vi "RT Main.vi"   [LabVIEW 2017]
doc: "This template is for the Queued Message Handler design pattern.\n\nThe Event Handling Loop generates messages based on user interface actions.\n\nThe Message Handling Loop processes messages generated by the Event Handling Loop, or by other messages. The messages are string values, so new messages can be added easily to the Message Cases case structure in the Message Handling Loop. Each message cluster can also provide an optional value for Message Data, which is a variant that can be converted to whatever message-specific data is required."
uses:
  controls/Functional Global Operation.ctl
  controls/Control State.ctl
  controls/Raw Values.ctl
  controls/Control Configuration.ctl
  Globals/Global - RT Stream Connections.vi
  Globals/Global - Configuration Options.vi
  support/Message Queue/Message Queue.lvlib
  <vilib>/nisyscfg/nisyscfg.lvlib
types:
  T1 = typedef "Functional Global Operation.ctl" = enum16{"Initialize", "Read", "Write"}
  T2 = typedef "Control State.ctl" = enum16{"Safe State", "Manual", "Control (PID)"}
  T3 = typedef "Raw Values.ctl" = cluster{"Channel 0":dbl, "Channel 1":dbl, "Channel 2":dbl, "Channel 3":dbl}
  T4 = typedef "Control Configuration.ctl" = cluster{"PID Gains":cluster{"proportional gain (Kc)":dbl, "integral gain (Kc*Ts/Ti)":dbl, "derivative gain (Kc*Td/Ts)":dbl}, "Output Range":cluster{"output high":dbl, "output low":dbl}}
  T5 = typedef "All Control Configuration Values.ctl" = cluster{"Control State":T2, "Setpoints":T3, "Manual Values":T3, "Control Configurations":T4[]}
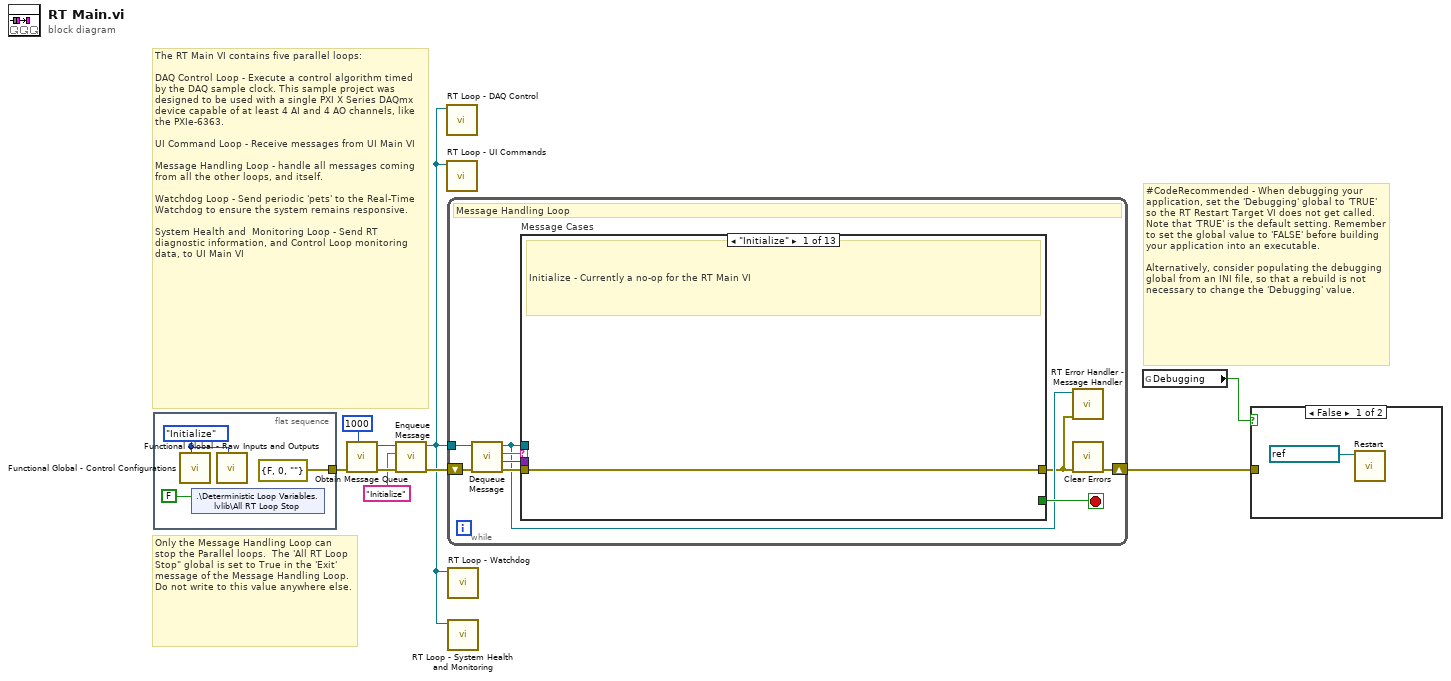
[diagram p0: block diagram]
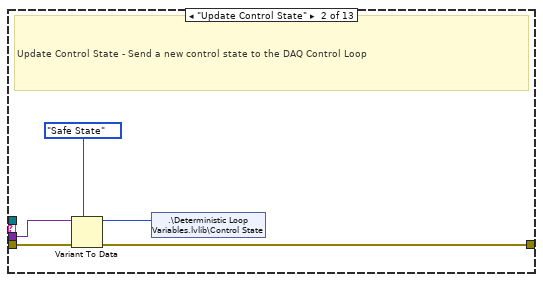
[diagram p3: hidden frame]
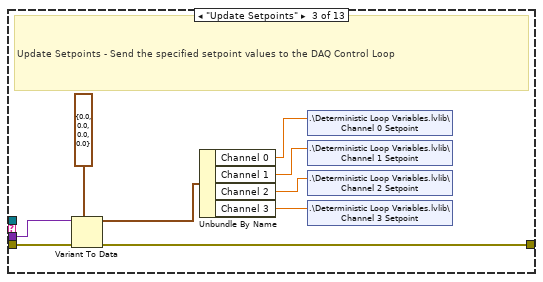
[diagram p4: hidden frame]
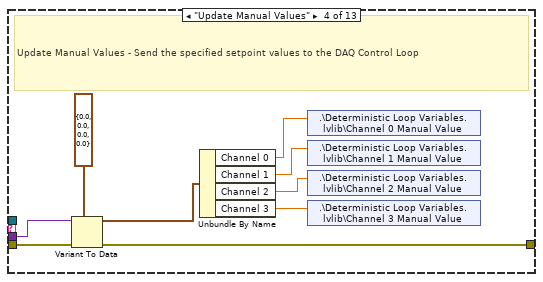
[diagram p5: hidden frame]
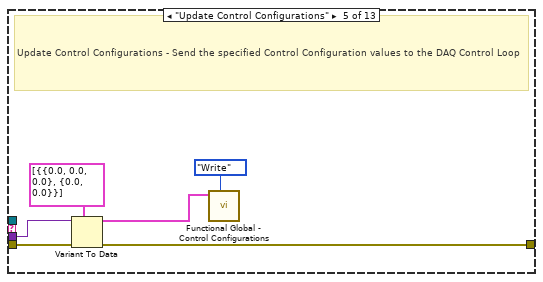
[diagram p6: hidden frame]
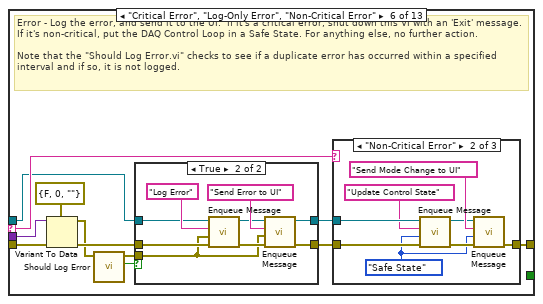
[diagram p7: hidden frame]
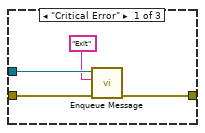
[diagram p9: hidden frame]
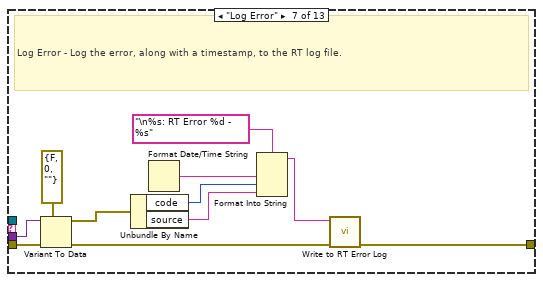
[diagram p11: hidden frame]
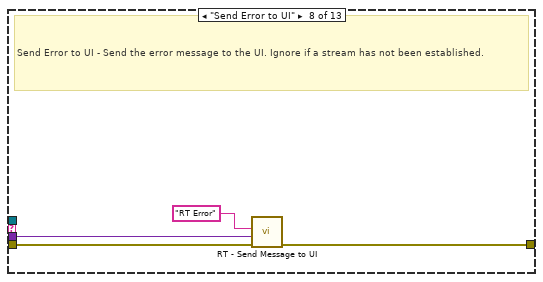
[diagram p12: hidden frame]
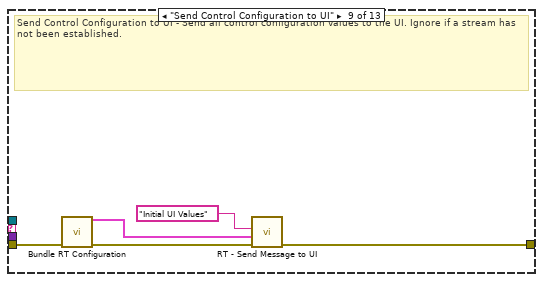
[diagram p13: hidden frame]
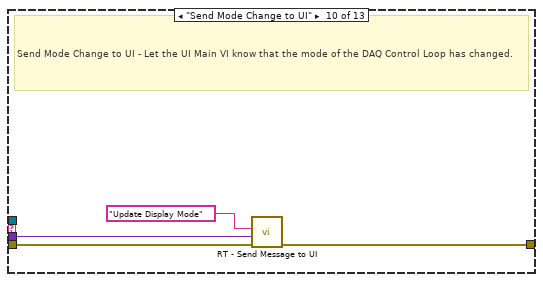
[diagram p14: hidden frame]
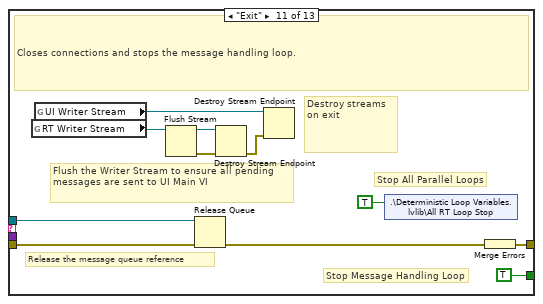
[diagram p15: hidden frame]
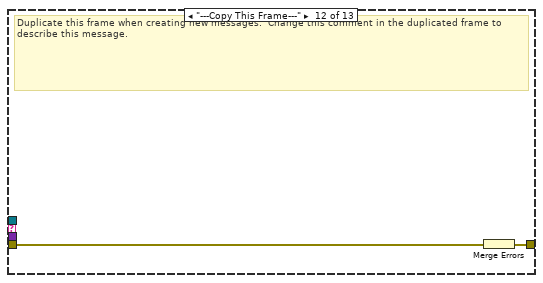
[diagram p16: hidden frame]
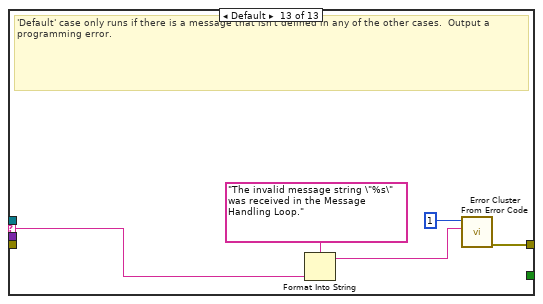
[diagram p17: hidden frame]
diagram:
  # "#CodeRecommended - When debugging your application, set the 'Debugging' global to 'TRUE' so the RT Restart Target VI does not get called.  Note that 'TRUE' is the default setting. Remember to set the global value to 'FALSE' before building your application into an executable.\n\nAlternatively, consider populating the debugging global from an INI file, so that a rebuild is not necessary to change the 'Debugging' value."
  # "The RT Main VI contains five parallel loops:\n\nDAQ Control Loop - Execute a control algorithm timed by the DAQ sample clock. This sample project was designed to be used with a single PXI X Series DAQmx device capable of at least 4 AI and 4 AO channels, like the PXIe-6363.\n\nUI Command Loop - Receive messages from UI Main VI\n\nMessage Handling Loop - handle all messages coming from all the other loops, and itself.\n\nWatchdog Loop - Send periodic 'pets' to the Real-Time Watchdog to ensure the system remains responsive.\n\nSystem Health and  Monitoring Loop - Send RT diagnostic information, and Control Loop monitoring data, to UI Main VI"
  # "Only the Message Handling Loop can stop the Parallel loops.  The 'All RT Loop Stop\" global is set to True in the 'Exit' message of the Message Handling Loop.  Do not write to this value anywhere else."
  n1 = flat-sequence {
    tunnel: [errorcluster {"status"=FALSE, "code"=0, "source"=""} ("error constant")] -> w4
    frame #0 {
      w10 = Functional_Global_Operation."Initialize" ("Functional Global Operation (Read)")
      n2 = call "Functional Global - Control Configurations.vi"("Functional Global Operation (Read)"=w10) -> ()  [unwired: 10 in, 1 out]
      n3 = shared-variable ".\\Deterministic Loop Variables.lvlib\\All RT Loop Stop"(FALSE) -> ()  [unwired: 1 in, 1 out]
      n4 = call "Functional Global - Raw Inputs and Outputs.vi"("Functional Global Operation (Read)"=w10) -> ()  [unwired: 9 in, 2 out]
    }
  }
  n5 = call "Obtain Message Queue.vi"("max queue size (-1, unlimited)"=1000, "error in (no error)"=w4) -> ("error out"=w9:errorcluster, "Message Queue"=w8:refnum<queue>)  [unwired: 8 in]
  n6 = call "Enqueue Message.vi"("error in (no error)"=w9, "Message"="Initialize", "Message Queue"=w8) -> ("error out"=w6:errorcluster, "dup Message Queue"=w2:refnum<queue>)  [unwired: 7 in]
  n7 = call "RT Loop - DAQ Control.vi"("Message Queue"=w2) -> ()  [unwired: 11 in]
  n8 = call "RT Loop - UI Commands.vi"("Message Queue"=w2) -> ()  [unwired: 11 in]
  n9 = while {
    tunnel: w2 -> [w16]
    shift-right: [w14] -> w3
    shift-left: w6 -> [w20]
    stop <- w21 stop-if-true
    # "Message Handling Loop"
    n10 = call "Dequeue Message.vi"("error in (no error)"=w20, "Message Queue"=w16) -> ("error out"=w19:errorcluster, "Message Data"=w17:variant, "Message"=w18:string, "dup Message Queue"=w15:refnum<queue>)  [unwired: 6 in]
    n11 = case "Message Cases" shown="\"Initialize\"" w18 {
      selector: w18 -> [_ _ _ _ _ w61 _ _ _ _ _ _ w128]
      tunnel: w15 -> [_ _ _ _ _ w55 _ _ _ _ w122 _ _]
      tunnel: w19 -> [w22 w27 w36 w45 w51 w59 w98 w102 w107 w111 w118 w124 _]
      tunnel: [w22 w24 w32 w41 w48 w60 w89 w99 w103 w110 w119 w123 w126] -> w13
      tunnel: [_ _ _ _ _ _ _ _ _ _ TRUE _ _] -> w21
      tunnel: w17 -> [_ w26 w35 w44 w50 w58 w97 w101 _ w109 _ _ _]
      frame "Initialize" {
        # "Initialize - Currently a no-op for the RT Main VI"
      }
      frame "Update Control State" {
        # "Update Control State - Send a new control state to the DAQ Control Loop"
        n12 = Variant To Data(error in=w27, type=Control_State."Safe State" ("FPGA State"), Variant=w26) -> (data=w23:T2, error out=w24:errorcluster)
        n13 = shared-variable ".\\Deterministic Loop Variables.lvlib\\Control State"(w23) -> ()  [unwired: 1 in, 1 out]
      }
      frame "Update Setpoints" {
        # "Update Setpoints - Send the specified setpoint values to the DAQ Control Loop"
        n14 = Variant To Data(error in=w36, type=T3 {"Channel 0"=0.0, "Channel 1"=0.0, "Channel 2"=0.0, "Channel 3"=0.0} ("Raw Values"), Variant=w35) -> (data=w33:T3, error out=w32:errorcluster)
        n15 = Unbundle By Name(w33) -> ("Channel 0"=w28:dbl, "Channel 1"=w29:dbl, "Channel 2"=w30:dbl, "Channel 3"=w31:dbl)
        n16 = shared-variable ".\\Deterministic Loop Variables.lvlib\\Channel 0 Setpoint"(w28) -> ()  [unwired: 1 in, 1 out]
        n17 = shared-variable ".\\Deterministic Loop Variables.lvlib\\Channel 1 Setpoint"(w29) -> ()  [unwired: 1 in, 1 out]
        n18 = shared-variable ".\\Deterministic Loop Variables.lvlib\\Channel 2 Setpoint"(w30) -> ()  [unwired: 1 in, 1 out]
        n19 = shared-variable ".\\Deterministic Loop Variables.lvlib\\Channel 3 Setpoint"(w31) -> ()  [unwired: 1 in, 1 out]
      }
      frame "Update Manual Values" {
        # "Update Manual Values - Send the specified setpoint values to the DAQ Control Loop"
        n20 = Variant To Data(error in=w45, type=T3 {"Channel 0"=0.0, "Channel 1"=0.0, "Channel 2"=0.0, "Channel 3"=0.0} ("Raw Values"), Variant=w44) -> (data=w42:T3, error out=w41:errorcluster)
        n21 = Unbundle By Name(w42) -> ("Channel 0"=w37:dbl, "Channel 1"=w38:dbl, "Channel 2"=w39:dbl, "Channel 3"=w40:dbl)
        n22 = shared-variable ".\\Deterministic Loop Variables.lvlib\\Channel 0 Manual Value"(w37) -> ()  [unwired: 1 in, 1 out]
        n23 = shared-variable ".\\Deterministic Loop Variables.lvlib\\Channel 1 Manual Value"(w38) -> ()  [unwired: 1 in, 1 out]
        n24 = shared-variable ".\\Deterministic Loop Variables.lvlib\\Channel 2 Manual Value"(w39) -> ()  [unwired: 1 in, 1 out]
        n25 = shared-variable ".\\Deterministic Loop Variables.lvlib\\Channel 3 Manual Value"(w40) -> ()  [unwired: 1 in, 1 out]
      }
      frame "Update Control Configurations" {
        # "Update Control Configurations - Send the specified Control Configuration values to the DAQ Control Loop"
        n26 = Variant To Data(error in=w51, type=T4[] [{"PID Gains"={"proportional gain (Kc)"=0.0, "integral gain (Kc*Ts/Ti)"=0.0, "derivative gain (Kc*Td/Ts)"=0.0}, "Output Range"={"output high"=0.0, "output low"=0.0}}], Variant=w50) -> (data=w47:T4[], error out=w48:errorcluster)
        n27 = call "Functional Global - Control Configurations.vi"("Functional Global Operation (Read)"=Functional_Global_Operation."Write", "Control Configurations in"=w47) -> ()  [unwired: 9 in, 1 out]
      }
      frame "Critical Error", "Log-Only Error", "Non-Critical Error" {
        # "Error - Log the error, and send it to the UI.  If it's a critical error, shut down this VI with an 'Exit' message. If it's non-critical, put the DAQ Control Loop in a Safe State. For anything else, no further action.\n\nNote that the \"Should Log Error.vi\" checks to see if a duplicate error has occurred within a specified interval and if so, it is not logged."
        n28 = Variant To Data(error in=w59, type=errorcluster {"status"=FALSE, "code"=0, "source"=""} ("error out"), Variant=w58) -> (data=w53:errorcluster, error out=w56:errorcluster)
        n29 = call "Should Log Error.vi"("error to report"=w53) -> ("Should Log Error?"=w54:bool, "dup error to report"=w52:errorcluster)  [unwired: 9 in]
        n30 = case shown="True" w54 {
          tunnel: [w65 w72] -> w63
          tunnel: [w64 w71] -> w62
          tunnel: w55 -> [w64 w70]
          tunnel: w56 -> [w65 w67]
          tunnel: w52 -> [_ w66]
          frame False {
          }
          frame True {
            n31 = call "Enqueue Message.vi"("error in (no error)"=w67, "Message Data"=w66, "Message"="Log Error", "Message Queue"=w70) -> ("error out"=w68:errorcluster, "dup Message Queue"=w69:refnum<queue>)  [unwired: 6 in]
            n32 = call "Enqueue Message.vi"("error in (no error)"=w68, "Message Data"=w66, "Message"="Send Error to UI", "Message Queue"=w69) -> ("error out"=w72:errorcluster, "dup Message Queue"=w71:refnum<queue>)  [unwired: 6 in]
          }
        }
        n33 = case shown="\"Non-Critical Error\"" w61 {
          tunnel: w63 -> [w78 w86 w87]
          tunnel: w62 -> [w76 w85 _]
          tunnel: [w77 w82 w87] -> w60
          frame "Critical Error" {
            n34 = call "Enqueue Message.vi"("error in (no error)"=w78, "Message"="Exit", "Message Queue"=w76) -> ("error out"=w77:errorcluster)  [unwired: 7 in, 1 out]
          }
          frame "Non-Critical Error" {
            w79 = Control_State."Safe State" ("FPGA State")
            n35 = call "Enqueue Message.vi"("error in (no error)"=w86, "Message Data"=w79, "Message"="Update Control State", "Message Queue"=w85) -> ("error out"=w83:errorcluster, "dup Message Queue"=w80:refnum<queue>)  [unwired: 6 in]
            n36 = call "Enqueue Message.vi"("error in (no error)"=w83, "Message Data"=w79, "Message"="Send Mode Change to UI", "Message Queue"=w80) -> ("error out"=w82:errorcluster)  [unwired: 6 in, 1 out]
          }
          frame Default {
          }
        }
      }
      frame "Log Error" {
        # "Log Error - Log the error, along with a timestamp, to the RT log file."
        n37 = Variant To Data(error in=w98, type=errorcluster {"status"=FALSE, "code"=0, "source"=""} ("error constant"), Variant=w97) -> (data=w92:errorcluster, error out=w95:errorcluster)
        n38 = Unbundle By Name(w92) -> ("code"=w91:i32, "source"=w90:string)
        n39 = Format Date/Time String() -> (date/time string=w93:string)  [unwired: 3 in]
        n40 = Format Into String(format string="\n%s: RT Error %d - %s", w93, w91, w90) -> (resulting string=w88:string)  [unwired: 2 in, 1 out]
        n41 = call "Write to RT Error Log.vi"("error in (no error)"=w95, "Log Entry"=w88) -> ("error out"=w89:errorcluster)  [unwired: 9 in]
      }
      frame "Send Error to UI" {
        # "Send Error to UI - Send the error message to the UI. Ignore if a stream has not been established."
        n42 = call "RT - Send Message to UI.vi"("error in (no error)"=w102, "Message Data"=w101, "Message"="RT Error") -> ("error out"=w99:errorcluster)  [unwired: 8 in]
      }
      frame "Send Control Configuration to UI" {
        # "Send Control Configuration to UI - Send all control configuration values to the UI. Ignore if a stream has not been established."
        n43 = call "Bundle RT Configuration.vi"("error in (no error)"=w107) -> ("error out"=w106:errorcluster, "All Control Configuration Values"=w105:T5)  [unwired: 9 in]
        n44 = call "RT - Send Message to UI.vi"("error in (no error)"=w106, "Message Data"=w105, "Message"="Initial UI Values") -> ("error out"=w103:errorcluster)  [unwired: 8 in]
      }
      frame "Send Mode Change to UI" {
        # "Send Mode Change to UI - Let the UI Main VI know that the mode of the DAQ Control Loop has changed."
        n45 = call "RT - Send Message to UI.vi"("error in (no error)"=w111, "Message Data"=w109, "Message"="Update Display Mode") -> ("error out"=w110:errorcluster)  [unwired: 8 in]
      }
      frame "Exit" {
        # "Flush the Writer Stream to ensure all pending messages are sent to UI Main VI"
        # "Destroy streams on exit"
        # "Stop Message Handling Loop"
        # "Stop All Parallel Loops"
        # "Release the message queue reference"
        # "Closes connections and stops the message handling loop."
        n46 = global read "Global - RT Stream Connections.vi" "RT Writer Stream"() -> (w117:refnum<k21>)
        n47 = global read "Global - RT Stream Connections.vi" "UI Writer Stream"() -> (w116:refnum<k21>)
        n48 = Flush Stream(11:w117) -> (0:w112:errorcluster, 3:w113:refnum<k21>)  [unwired: 3 in, 1 out]
        n49 = Release Queue(queue=w122, error in (no error)=w118) -> (error out=w120:errorcluster)  [unwired: 1 in, 2 out]
        n50 = Destroy Stream Endpoint(8:w112, 11:w113) -> (0:w115:errorcluster)
        n51 = Destroy Stream Endpoint(8:w115, 11:w116) -> ()  [unwired: 1 out]
        n52 = shared-variable ".\\Deterministic Loop Variables.lvlib\\All RT Loop Stop"(TRUE ("Stop Monitoring Loops")) -> ()  [unwired: 1 in, 1 out]
        n53 = Merge Errors(w120) -> (w119:errorcluster)
      }
      frame "---Copy This Frame---" {
        # "Duplicate this frame when creating new messages.  Change this comment in the duplicated frame to describe this message."
        n54 = Merge Errors(w124) -> (w123:errorcluster)
      }
      frame Default {
        # "'Default' case only runs if there is a message that isn't defined in any of the other cases.  Output a programming error."
        n55 = Format Into String(format string="The invalid message string \"%s\" was received in the Message Handling Loop." ("Unknown Message Error Text"), w128) -> (resulting string=w125:string)  [unwired: 2 in, 1 out]
        n56 = call <vilib>:"Error Cluster From Error Code.vi"("error message (\"\")"=w125, "error code (0)"=1) -> ("error out"=w126:errorcluster)  [unwired: 7 in]
      }
    }
    n57 = call "RT Error Handler - Message Handler.vi"("error in (no error)"=w13, "Message Queue"=w15) -> ()  [unwired: 9 in, 1 out]
    n58 = call <vilib>:"Clear Errors.vi"("error in (no error)"=w13) -> ("error out"=w14:errorcluster)  [unwired: 5 in, 1 out]
  }
  n59 = call "RT Loop - Watchdog.vi"("Message Queue"=w2) -> ()  [unwired: 11 in]
  n60 = call "RT Loop - System Health and Monitoring.vi"("Message Queue"=w2) -> ()  [unwired: 11 in]
  n61 = global read "Global - Configuration Options.vi" "Debugging"() -> (w5:bool)
  n62 = case shown="False" w5 {
    tunnel: w3 -> [_ _]
    frame False {
      n63 = call <vilib>:"Restart.vi"("Session in"=refnum<k21> "localhost" ("session in")) -> ()  [unwired: 8 in, 3 out]
    }
    frame True {
    }
  }
